vi "Sensor Display.vi"(5 "sensors":T3={"net distance (mm)"=0, "net angle (deg)"=0, "accelerometer"={"x axis (g)"=0.0, "y axis (g)"=0.0, "z axis (g)"=0.0}, "iRobot Sensors"={"Bumps + Wheel Drops"={"Wheeldrop Caster"=FALSE, "Wheeldrop Left"=FALSE, "Wheeldrop Right"=FALSE, "Bump Left"=FALSE, "Bump Right"=FALSE}, "Wall"=FALSE, "Cliff Left"=FALSE, "Cliff Front Left"=FALSE, "Cliff Front Right"=FALSE, "Cliff Right"=FALSE, "Wall Signal"=0, "Cliff Left Signal"=0, "Cliff Front Left Signal"=0, "Cliff Front Right Signal"=0, "Cliff Right Signal"=0, "Buttons"={"Advance"=FALSE, "Play"=FALSE}, "Virtual Wall"=FALSE, "# Stream Packets"=0, "Requested Velocity (mm/s)"=0, "Requested Radius (mm)"=0, "Requested Right Wheel Velocity (mm/s)"=0, "Requested Left Wheel Velocity (mm/s)"=0, "Distance (mm)"=0, "Angle (deg)"=0, "Song Playing"=FALSE, "Song Number"=0, "Charging State"=enum."Not Charging", "Voltage (mV)"=0, "Current (mA)"=0, "Battery Temperature (deg C)"=0, "Battery Charge (mAh)"=0, "Battery Capacity (mAh)"=0, "Charging Sources"={"Internal Charger"=FALSE, "Home Base"=FALSE}, "OI Mode"=enum."Off", "Digital Inputs"={"Digital Input 0"=FALSE, "Digital Input 1"=FALSE, "Digital Input 2"=FALSE, "Digital Input 3"=FALSE, "Device Detect"=FALSE}, "Drivers & Wheel Overcurrent"={"Low-Side Driver 0"=FALSE, "Low-Side Driver 1"=FALSE, "Low-Side Driver 2"=FALSE, "Left Wheel"=FALSE, "Right Wheel"=FALSE}, "Analog Signal"=0, "Infrared"=255}, "Is Simulator?"=FALSE, "Kobuki Sensors"={"Bumps + Wheel Drops"={"Wheeldrop Left"=FALSE, "Wheeldrop Right"=FALSE, "Bump Left"=FALSE, "Bump Center"=FALSE, "Bump Right"=FALSE}, "Cliff Left"=FALSE, "Cliff Center"=FALSE, "Cliff Right"=FALSE, "Cliff Left Signal"=0, "Cliff Center Signal"=0, "Cliff Right Signal"=0, "Buttons"={"B0"=FALSE, "B1"=FALSE, "B2"=FALSE}, "# Stream Packets"=0, "Requested Velocity (mm/s)"=0, "Requested Radius (mm)"=0, "Requested Right Wheel Velocity (mm/s)"=0, "Requested Left Wheel Velocity (mm/s)"=0, "Left Wheel Encoder (ticks)"=0, "Angle (deg)"=0, "Song Playing"=FALSE, "Song Number"=0, "Charging State"=enum."Not Charging", "Voltage (mV)"=0, "Current (mA)"=0, "Battery Temperature (deg C)"=0, "Battery Charge (mAh)"=0, "Battery Capacity (mAh)"=0, "Charging Sources"={"Internal Charger"=FALSE, "Home Base"=FALSE}, "OI Mode"=enum."Off", "Digital Inputs"={"Digital Input 0"=FALSE, "Digital Input 1"=FALSE, "Digital Input 2"=FALSE, "Digital Input 3"=FALSE, "Device Detect"=FALSE}, "Drivers & Wheel Overcurrent"={"Low-Side Driver 0"=FALSE, "Low-Side Driver 1"=FALSE, "Low-Side Driver 2"=FALSE, "Left Wheel"=FALSE, "Right Wheel"=FALSE}, "Analog Signal"=0, "Infrared"=255, "Right Wheel Encoder (ticks) "=0, "TimeStamp"=0}} {"Kobuki Sensors"."Infrared" format="%02x"; "iRobot Sensors"."Infrared" format="%02x"; "accelerometer"."z axis (g)" format="%.3f"; "accelerometer"."y axis (g)" format="%.3f"; "accelerometer"."x axis (g)" format="%.3f"}) -> (2 "irobot sensor display":T1 {"Right Wheel (mm/s)" scale=-500.0..500.0; "Left Wheel (mm/s)" scale=-500.0..500.0})   [LabVIEW 2014]
doc: "Convert robot sensors into a graphical control for display in UI."
uses:
  Sensors.ctl
  iRobot/Sensor/Accelerometer.ctl
  iRobot/Sensor/Sensor Group 6.ctl
  iRobot/Sensor/Bumps + Wheel Drops.ctl
  iRobot/Sensor/Buttons.ctl
  iRobot/Sensor/Charging State.ctl
  iRobot/Sensor/Charging Sources Available.ctl
  iRobot/Sensor/OI Mode.ctl
  iRobot/Sensor/Cargo Bay Digital Inputs.ctl
  iRobot/Sensor/Low-Side Driver + Wheel Overcurrent.ctl
  Kobuki/KobukiSensors.ctl
  Kobuki/Kobuki Bumps and WheelDrops.ctl
  Kobuki/Kobuki Buttons.ctl
  iRobot Sensor Display.ctl
panel:
  # "Electrical: charging, battery, OI mode"
  # "Sensors: bump, cliff, button, wheel drop, wall, virtual wall"
  # "Motion: distance, angle, requested velocity"
  # "Cargo Bay: I/O, overcurrent, infrared"
  # "Song"
  # "Electrical: charging, battery, OI mode"
  # "Sensors: bump, cliff, button, wheel drop, wall, virtual wall"
  # "Motion: distance, angle, requested velocity"
  # "Cargo Bay: I/O, overcurrent, infrared"
  # "Song"
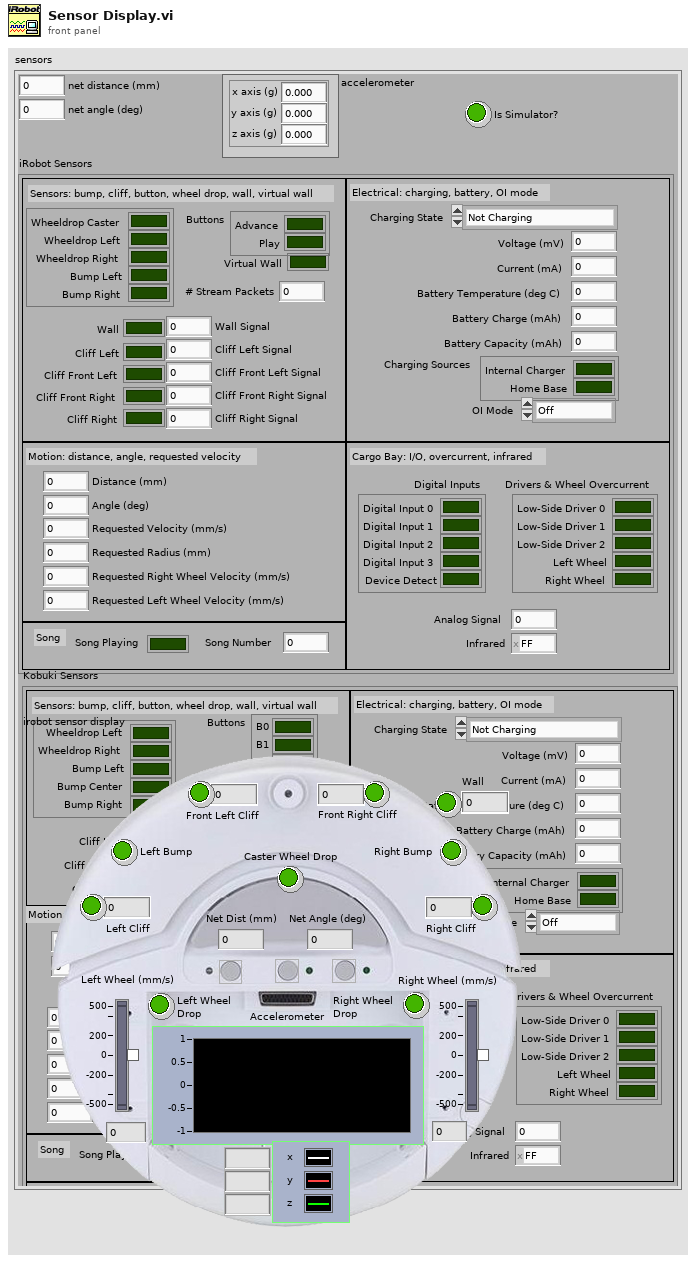
[diagram p1: front panel]
types:
  T1 = typedef "iRobot Sensor Display.ctl" = cluster{"Caster Wheel Drop":bool, "Left Wheel\nDrop":bool, "Right Wheel \nDrop":bool, "Left Bump":bool, "Right Bump":bool, "Left Cliff":bool, "Front Left Cliff":bool, "Front Right Cliff":bool, "Right Cliff":bool, "Wall":bool, "Net Dist (mm)":i32, "Net Angle (deg)":i32, "Wall":u16, "Left Cliff":u16, "Front Left Cliff":u16, "Front Right Cliff":u16, "Right Cliff":u16, "Left Wheel (mm/s)":i16, "Right Wheel (mm/s)":i16, "Accelerometer":T2}
  T2 = typedef "Accelerometer.ctl" = cluster{"x axis (g)":dbl, "y axis (g)":dbl, "z axis (g)":dbl}
  T3 = typedef "Sensors.ctl" = cluster{"net distance (mm)":i32, "net angle (deg)":i32, "accelerometer":T2, "iRobot Sensors":T4, "Is Simulator?":bool, "Kobuki Sensors":T12}
  T4 = typedef "Sensor Group 6.ctl" = cluster{"Bumps + Wheel Drops":T5, "Wall":bool, "Cliff Left":bool, "Cliff Front Left":bool, "Cliff Front Right":bool, "Cliff Right":bool, "Wall Signal":u16, "Cliff Left Signal":u16, "Cliff Front Left Signal":u16, "Cliff Front Right Signal":u16, "Cliff Right Signal":u16, "Buttons":T6, "Virtual Wall":bool, "# Stream Packets":u8, "Requested Velocity (mm/s)":i16, "Requested Radius (mm)":i16, "Requested Right Wheel Velocity (mm/s)":i16, "Requested Left Wheel Velocity (mm/s)":i16, "Distance (mm)":i32, "Angle (deg)":i32, "Song Playing":bool, "Song Number":u8, "Charging State":T7, "Voltage (mV)":u16, "Current (mA)":i16, "Battery Temperature (deg C)":i8, "Battery Charge (mAh)":u16, "Battery Capacity (mAh)":u16, "Charging Sources":T8, "OI Mode":T9, "Digital Inputs":T10, "Drivers & Wheel Overcurrent":T11, "Analog Signal":u16, "Infrared":u8}
  T5 = typedef "Bumps + Wheel Drops.ctl" = cluster{"Wheeldrop Caster":bool, "Wheeldrop Left":bool, "Wheeldrop Right":bool, "Bump Left":bool, "Bump Right":bool}
  T6 = typedef "Buttons.ctl" = cluster{"Advance":bool, "Play":bool}
  T7 = typedef "Charging State.ctl" = enum16{"Not Charging", "Reconditioning Charging", "Full Charging", "Trickle Charging", "Waiting", "Charging Fault Condition"}
  T8 = typedef "Charging Sources Available.ctl" = cluster{"Internal Charger":bool, "Home Base":bool}
  T9 = typedef "OI Mode.ctl" = enum16{"Off", "Passive", "Safe", "Full"}
  T10 = typedef "Cargo Bay Digital Inputs.ctl" = cluster{"Digital Input 0":bool, "Digital Input 1":bool, "Digital Input 2":bool, "Digital Input 3":bool, "Device Detect":bool}
  T11 = typedef "Low-Side Driver + Wheel Overcurrent.ctl" = cluster{"Low-Side Driver 0":bool, "Low-Side Driver 1":bool, "Low-Side Driver 2":bool, "Left Wheel":bool, "Right Wheel":bool}
  T12 = typedef "KobukiSensors.ctl" = cluster{"Bumps + Wheel Drops":T13, "Cliff Left":bool, "Cliff Center":bool, "Cliff Right":bool, "Cliff Left Signal":u16, "Cliff Center Signal":u16, "Cliff Right Signal":u16, "Buttons":T14, "# Stream Packets":u8, "Requested Velocity (mm/s)":i16, "Requested Radius (mm)":i16, "Requested Right Wheel Velocity (mm/s)":i16, "Requested Left Wheel Velocity (mm/s)":i16, "Left Wheel Encoder (ticks)":i16, "Angle (deg)":i32, "Song Playing":bool, "Song Number":u8, "Charging State":T7, "Voltage (mV)":u16, "Current (mA)":i16, "Battery Temperature (deg C)":i8, "Battery Charge (mAh)":u16, "Battery Capacity (mAh)":u16, "Charging Sources":T8, "OI Mode":T9, "Digital Inputs":T10, "Drivers & Wheel Overcurrent":T11, "Analog Signal":u16, "Infrared":u8, "Right Wheel Encoder (ticks) ":i16, "TimeStamp":u16}
  T13 = typedef "Kobuki Bumps and WheelDrops.ctl" = cluster{"Wheeldrop Left":bool, "Wheeldrop Right":bool, "Bump Left":bool, "Bump Center":bool, "Bump Right":bool}
  T14 = typedef "Kobuki Buttons.ctl" = cluster{"B0":bool, "B1":bool, "B2":bool}
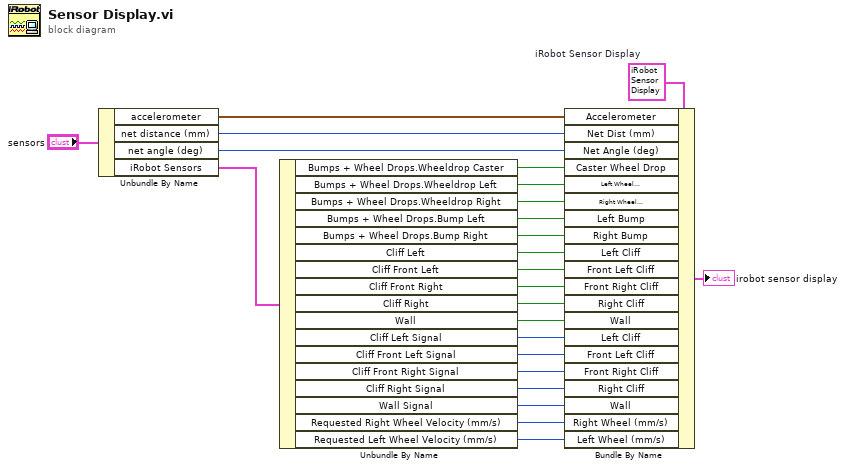
[diagram p0: block diagram]
diagram:
  w4 = T1 {"Caster Wheel Drop"=FALSE, "Left Wheel\nDrop"=FALSE, "Right Wheel \nDrop"=FALSE, "Left Bump"=FALSE, "Right Bump"=FALSE, "Left Cliff"=FALSE, "Front Left Cliff"=FALSE, "Front Right Cliff"=FALSE, "Right Cliff"=FALSE, "Wall"=FALSE, "Net Dist (mm)"=0, "Net Angle (deg)"=0, "Wall"=0, "Left Cliff"=0, "Front Left Cliff"=0, "Front Right Cliff"=0, "Right Cliff"=0, "Left Wheel (mm/s)"=0, "Right Wheel (mm/s)"=0, "Accelerometer"={"x axis (g)"=0.0, "y axis (g)"=0.0, "z axis (g)"=0.0}}  # iRobot Sensor Display
  n1 = Unbundle By Name("sensors") -> ("accelerometer"=w6:T2, "net distance (mm)"=w7:i32, "net angle (deg)"=w8:i32, "iRobot Sensors"=w9:T4)
  n2 = Unbundle By Name(w9) -> ("Bumps + Wheel Drops.Wheeldrop Caster"=w24:bool, "Bumps + Wheel Drops.Wheeldrop Left"=w23:bool, "Bumps + Wheel Drops.Wheeldrop Right"=w22:bool, "Bumps + Wheel Drops.Bump Left"=w21:bool, "Bumps + Wheel Drops.Bump Right"=w20:bool, "Cliff Left"=w19:bool, "Cliff Front Left"=w18:bool, "Cliff Front Right"=w17:bool, "Cliff Right"=w16:bool, "Wall"=w15:bool, "Cliff Left Signal"=w14:u16, "Cliff Front Left Signal"=w13:u16, "Cliff Front Right Signal"=w12:u16, "Cliff Right Signal"=w11:u16, "Wall Signal"=w10:u16, "Requested Right Wheel Velocity (mm/s)"=w2:i16, "Requested Left Wheel Velocity (mm/s)"=w1:i16)
  n3 = Bundle By Name(cluster=w4, "Accelerometer"=w6, "Net Dist (mm)"=w7, "Net Angle (deg)"=w8, "Caster Wheel Drop"=w24, "Left Wheel\nDrop"=w23, "Right Wheel \nDrop"=w22, "Left Bump"=w21, "Right Bump"=w20, "Left Cliff"=w19, "Front Left Cliff"=w18, "Front Right Cliff"=w17, "Right Cliff"=w16, "Wall"=w15, "Left Cliff"=w14, "Front Left Cliff"=w13, "Front Right Cliff"=w12, "Right Cliff"=w11, "Wall"=w10, "Right Wheel (mm/s)"=w2, "Left Wheel (mm/s)"=w1) -> (→"irobot sensor display":T1)
